vi "clean_cycle.vi"(11 "seconds to wait":u32=8) -> ()   [LabVIEW 2016]
panel:
  out "ms to wait":u32=7000
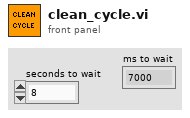
[diagram p1: front panel]
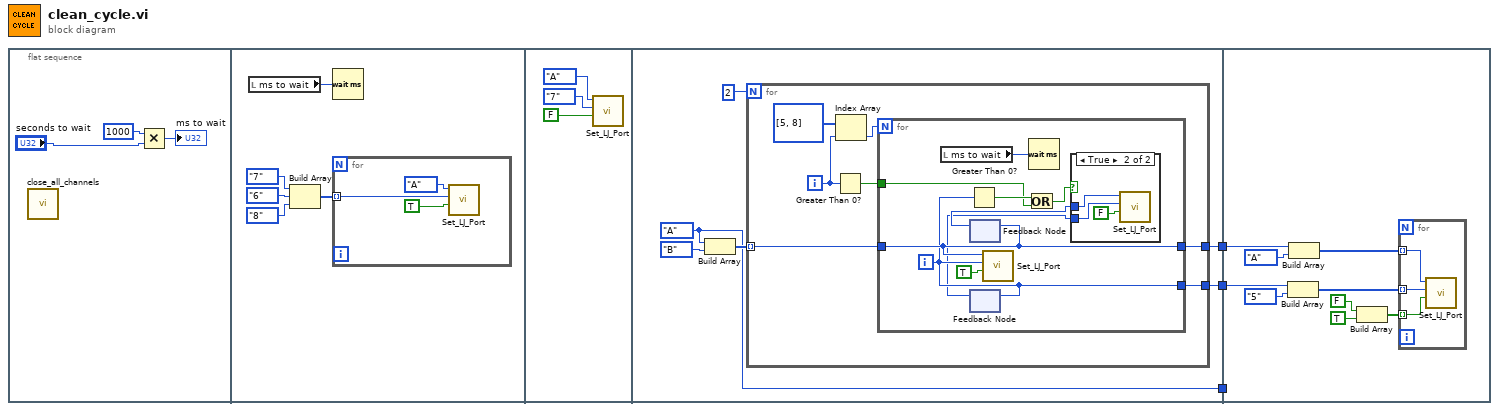
[diagram p0: block diagram]
diagram:
  n1 = flat-sequence {
    tunnel: [w20] -> w3
    tunnel: [w19] -> w2
    tunnel: [w18] -> w1
    tunnel: w3 -> [_]
    tunnel: w2 -> [w48]
    tunnel: w1 -> [w47]
    frame #0 {
      n2 = call "close_all_channels.vi"() -> ()  [unwired: 12 in]
      n3 = Multiply(x=u32 1000, y="seconds to wait") -> (x*y=→"ms to wait":u32)
    }
    frame #1 {
      n4 = local read "ms to wait"() -> (w7:u32)
      n5 = Build Array(enum16{"1", "2", "3", "4", "5", "6", "7", "8"}."7" ("Channel"), enum16{"1", "2", "3", "4", "5", "6", "7", "8"}."6" ("Channel"), enum16{"1", "2", "3", "4", "5", "6", "7", "8"}."8" ("Channel")) -> (w11:enum16{"1", "2", "3", "4", "5", "6", "7", "8"}[])
      n6 = Wait (ms)(milliseconds to wait=w7) -> ()  [unwired: 1 out]
      n7 = for {
        tunnel: w11 -> [w14] mode=indexing
        n8 = call "Set_LJ_Port.vi"("State"=TRUE, "Channel"=w14, "Flowboard"=enum16{"A", "B", "C"}."A") -> ()  [unwired: 8 in, 1 out]
      }
    }
    frame #2 {
      n9 = call "Set_LJ_Port.vi"("State"=FALSE, "Channel"=enum16{"1", "2", "3", "4", "5", "6", "7", "8"}."7", "Flowboard"=enum16{"A", "B", "C"}."A") -> ()  [unwired: 8 in, 1 out]
    }
    frame #3 {
      w20 = enum16{"A", "B", "C"}."A" ("Flowboard")
      n10 = Build Array(w20, enum16{"A", "B", "C"}."B" ("Flowboard")) -> (w23:enum16{"A", "B", "C"}[])
      n11 = for {
        N: 2 -> [_]
        tunnel: w23 -> [w28] mode=indexing
        tunnel: [w27] -> w19
        tunnel: [w26] -> w18
        i -> [w25]
        n12 = Greater Than 0?(x=w25) -> (x > 0?=w24:bool)
        n13 = Index Array(array=i32[] [5, 8], index=w25) -> (element=w29:i32)
        n14 = for {
          N: w29 -> [_]
          tunnel: w28 -> [w38]
          tunnel: [w38] -> w27
          tunnel: [w37] -> w26
          tunnel: w24 -> [w35]
          i -> [w37]
          n15 = local read "ms to wait"() -> (w31:u32)
          n16 = Greater Than 0?(x=w37) -> (x > 0?=w36:bool)
          n17 = feedback #1() -> (w34:enum16{"A", "B", "C"})  [unwired: 1 in]
          n18 = feedback-in #1(w38) -> ()
          n19 = feedback #2() -> (w33:i32)  [unwired: 1 in]
          n20 = feedback-in #2(w37) -> ()
          n21 = call "Set_LJ_Port.vi"("State"=TRUE, "Channel"=w37, "Flowboard"=w38) -> ()  [unwired: 8 in, 1 out]
          n22 = Or(x=w36, y=w35) -> (x .or. y?=w32:bool)
          n23 = Wait (ms)(milliseconds to wait=w31) -> ()  [unwired: 1 out]
          n24 = case shown="True" w32 {
            tunnel: w34 -> [_ w42]
            tunnel: w33 -> [_ w41]
            frame False {
            }
            frame True {
              n25 = call "Set_LJ_Port.vi"("State"=FALSE, "Channel"=w41, "Flowboard"=w42) -> ()  [unwired: 8 in, 1 out]
            }
          }
        }
      }
    }
    frame #4 {
      n26 = Build Array(w47, enum16{"1", "2", "3", "4", "5", "6", "7", "8"}."5" ("Channel")) -> (w43:i32[])
      n27 = Build Array(w48, enum16{"A", "B", "C"}."A" ("element")) -> (w44:enum16{"A", "B", "C"}[])
      n28 = Build Array(FALSE ("State"), TRUE ("State")) -> (w49:bool[])
      n29 = for {
        tunnel: w49 -> [w54] mode=indexing
        tunnel: w44 -> [w53] mode=indexing
        tunnel: w43 -> [w52] mode=indexing
        n30 = call "Set_LJ_Port.vi"("State"=w54, "Channel"=w52, "Flowboard"=w53) -> ()  [unwired: 8 in, 1 out]
      }
    }
  }
